vi "init Power Supply.vi"(9 "devID":u32, 10 "name":string, 11 "mds":string) -> (1 "devID out":u32, 3 "function return":i32)   [LabVIEW 2014, in "libchaos-driver-powersupply-labview.lvlib"]
doc: "int initPowerSupply(const char* mds,const char* name, unsigned int* devID);"
uses:
  libchaos-driver-powersupply-labview.lvlib
  chaos-i686-dynamic-release/lib/libchaos-driver-powersupply-labview.so
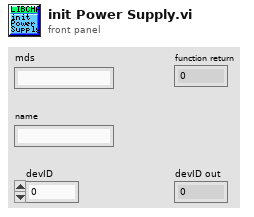
[diagram p1: front panel]
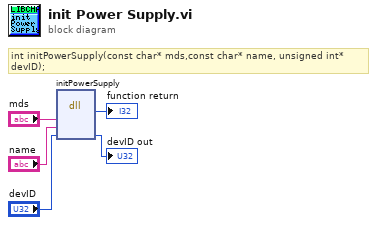
[diagram p0: block diagram]
diagram:
  # "int initPowerSupply(const char* mds,const char* name, unsigned int* devID);"
  n1 = dll-call lib="home/chaos/chaos_bundle/chaos-i686-dynamic-release/lib/libchaos-driver-powersupply-labview.*" fn="initPowerSupply"("mds"="mds", "name"="name", "devID"="devID") -> (→"function return":i32, "devID"=→"devID out":u32)  [unwired: 5 in, 2 out]
